vi "Get_Create_Gserver_SettingsPath.vi"(8 "error in (no error)":errorcluster, 9 "ViewPortName":string, 11 "Gserver in":refnum<class "Gserver.lvclass">) -> (0 "error out":errorcluster, 1 "Viewport settings path":path, 3 "Gserver out":refnum<class "Gserver.lvclass">)   [LabVIEW 2020, in "Gserver.lvclass"]
doc: "Andre Koelewijn, 3 jan 2021\n\nProvide and/or create the folder location where the Gviewer graph application can store and retrieve the specific graph settings of the viewport with that name."
uses:
  Gserver.lvclass
  Gserver.lvclass/Gserver.ctl
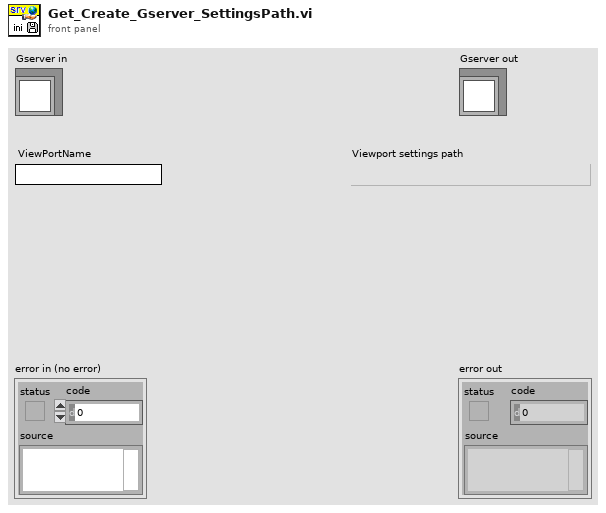
[diagram p1: front panel]
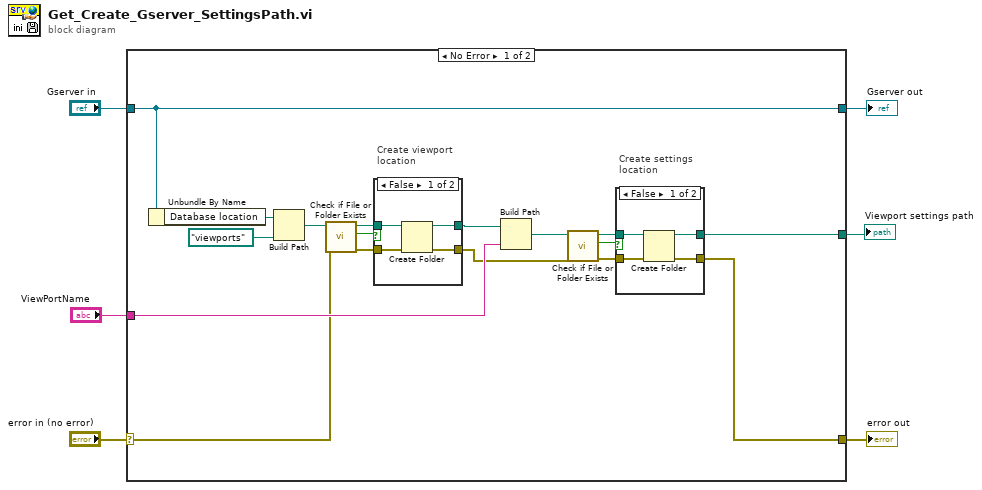
[diagram p0: block diagram]
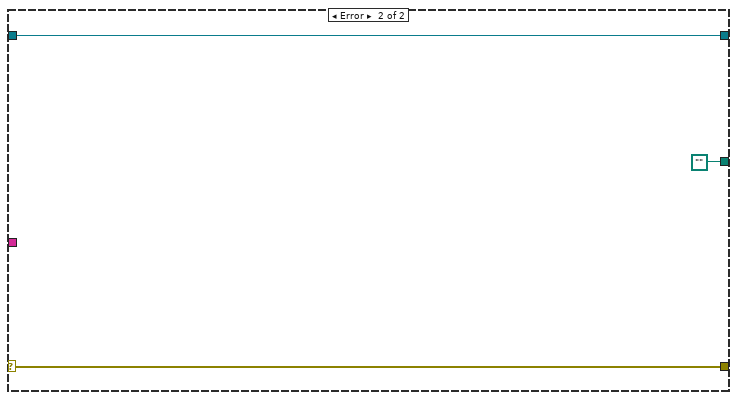
[diagram p4: hidden frame]
diagram:
  n1 = case shown="No Error" "error in (no error)" {
    selector: "error in (no error)" -> [w9 w38]
    tunnel: [w8 w38] -> w5
    tunnel: [w23 w37] -> w3
    tunnel: "Gserver in" -> [w23 w37]
    tunnel: "ViewPortName" -> [w15 _]
    tunnel: [w7 path ""] -> w1
    frame No Error {
      # "Create settings\nlocation"
      # "Create viewport\nlocation"
      n2 = Unbundle By Name(w23) -> ("Database location"=w22:path)
      n3 = Build Path(base path=w22, name or relative path=path "viewports") -> (appended path=w20:path)
      n4 = call <vilib>:"Check if File or Folder Exists.vi"("error in (no error)"=w9, "path"=w20) -> ("error out"=w18:errorcluster, "file or folder exists?"=w19:bool, "dup path"=w17:path)  [unwired: 7 in]
      n5 = case shown="False" w19 {
        tunnel: w18 -> [w33 w34]
        tunnel: w17 -> [w32 w35]
        tunnel: [w31 w34] -> w10
        tunnel: [w30 w35] -> w16
        frame False {
          n6 = Create Folder(path (use dialog)=w32, error in=w33) -> (created path=w30:path, error out=w31:errorcluster)  [unwired: 1 in, 1 out]
        }
        frame True {
        }
      }
      n7 = Build Path(base path=w16, name or relative path=w15) -> (appended path=w11:path)
      n8 = call <vilib>:"Check if File or Folder Exists.vi"("error in (no error)"=w10, "path"=w11) -> ("error out"=w13:errorcluster, "file or folder exists?"=w12:bool, "dup path"=w14:path)  [unwired: 7 in]
      n9 = case shown="False" w12 {
        tunnel: w13 -> [w27 w28]
        tunnel: w14 -> [w26 w29]
        tunnel: [w25 w28] -> w8
        tunnel: [w24 w29] -> w7
        frame False {
          n10 = Create Folder(path (use dialog)=w26, error in=w27) -> (created path=w24:path, error out=w25:errorcluster)  [unwired: 1 in, 1 out]
        }
        frame True {
        }
      }
    }
    frame Error {
    }
  }
  "error out" <- w5
  "Gserver out" <- w3
  "Viewport settings path" <- w1
